vi "Main.vi"() -> ()   [LabVIEW 2023]
uses:
  Control/Time.ctl
panel:
  in  "stop":bool
  out "ms":dbl
  in  "碼表":bool
  in  "時鐘":bool
  in  "Tab Control":enum32{"Page 1", "Page 2"}(tab)
  out "Alarm Photo":picture
  out "Needle":cluster{dbl[], dbl[]}[](graph)
  out "clock":picture
  out "TIme":T1
  in  "Set Time":bool
  in  "Set second":i32(knob) scale=0.0..60.0
  in  "Set minute":i32(knob) scale=0.0..60.0
  in  "Set hour":i32(knob) scale=0.0..24.0
  in  "Set Alarm":bool
  in  "鬧鐘時間":timestamp format="%<%H:%M>T"
  in  "鬧鐘模式":u16(ring) items=["聲音模式", "畫面模式"]
  in  "Alarm Sound Path":path
  in  "Alarm Photo Path":path
  in  "開始/暫停碼表":bool
  in  "重置碼表":bool
  out "碼表時間":dbl
  out "碼表":i16(knob) scale=0.0..60.0
  out "smile":picture
  out "pi/180":dbl
  # "時"
  # "分"
  # "秒"
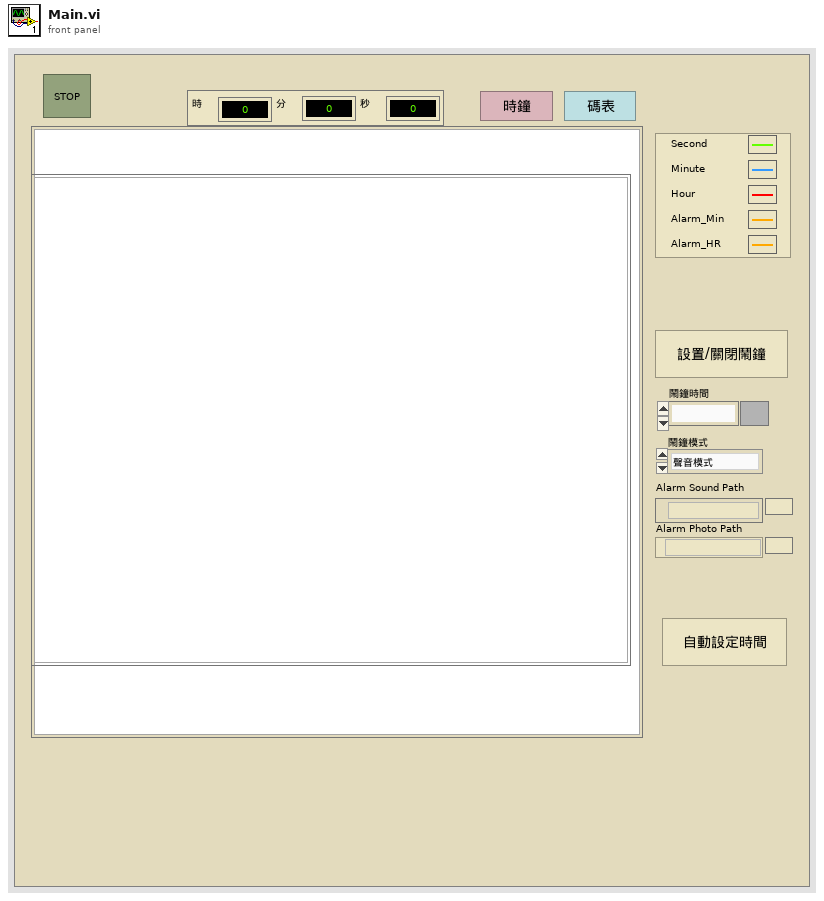
[diagram p1: front panel]
types:
  T1 = typedef "Time.ctl" = cluster{"hour":i32, "minute":i32, "second":i32}
  T2 = typedef "LVDateTimeRec.ctl" = cluster{"fractional second":dbl, "second":i32, "minute":i32, "hour":i32, "day of month":i32, "month":i32, "year":i32, "day of week":i32, "day of year":i32, "DST":i32}
  T3 = typedef "Sound Output Task ID.ctl" = u32
  T4 = typedef "imagedata.ctl" = cluster{"image type":i32, "image depth":i32, "image":u8[], "mask":u8[], "colors":u32[], "Rectangle":cluster{"left":i16, "top":i16, "right":i16, "bottom":i16}}
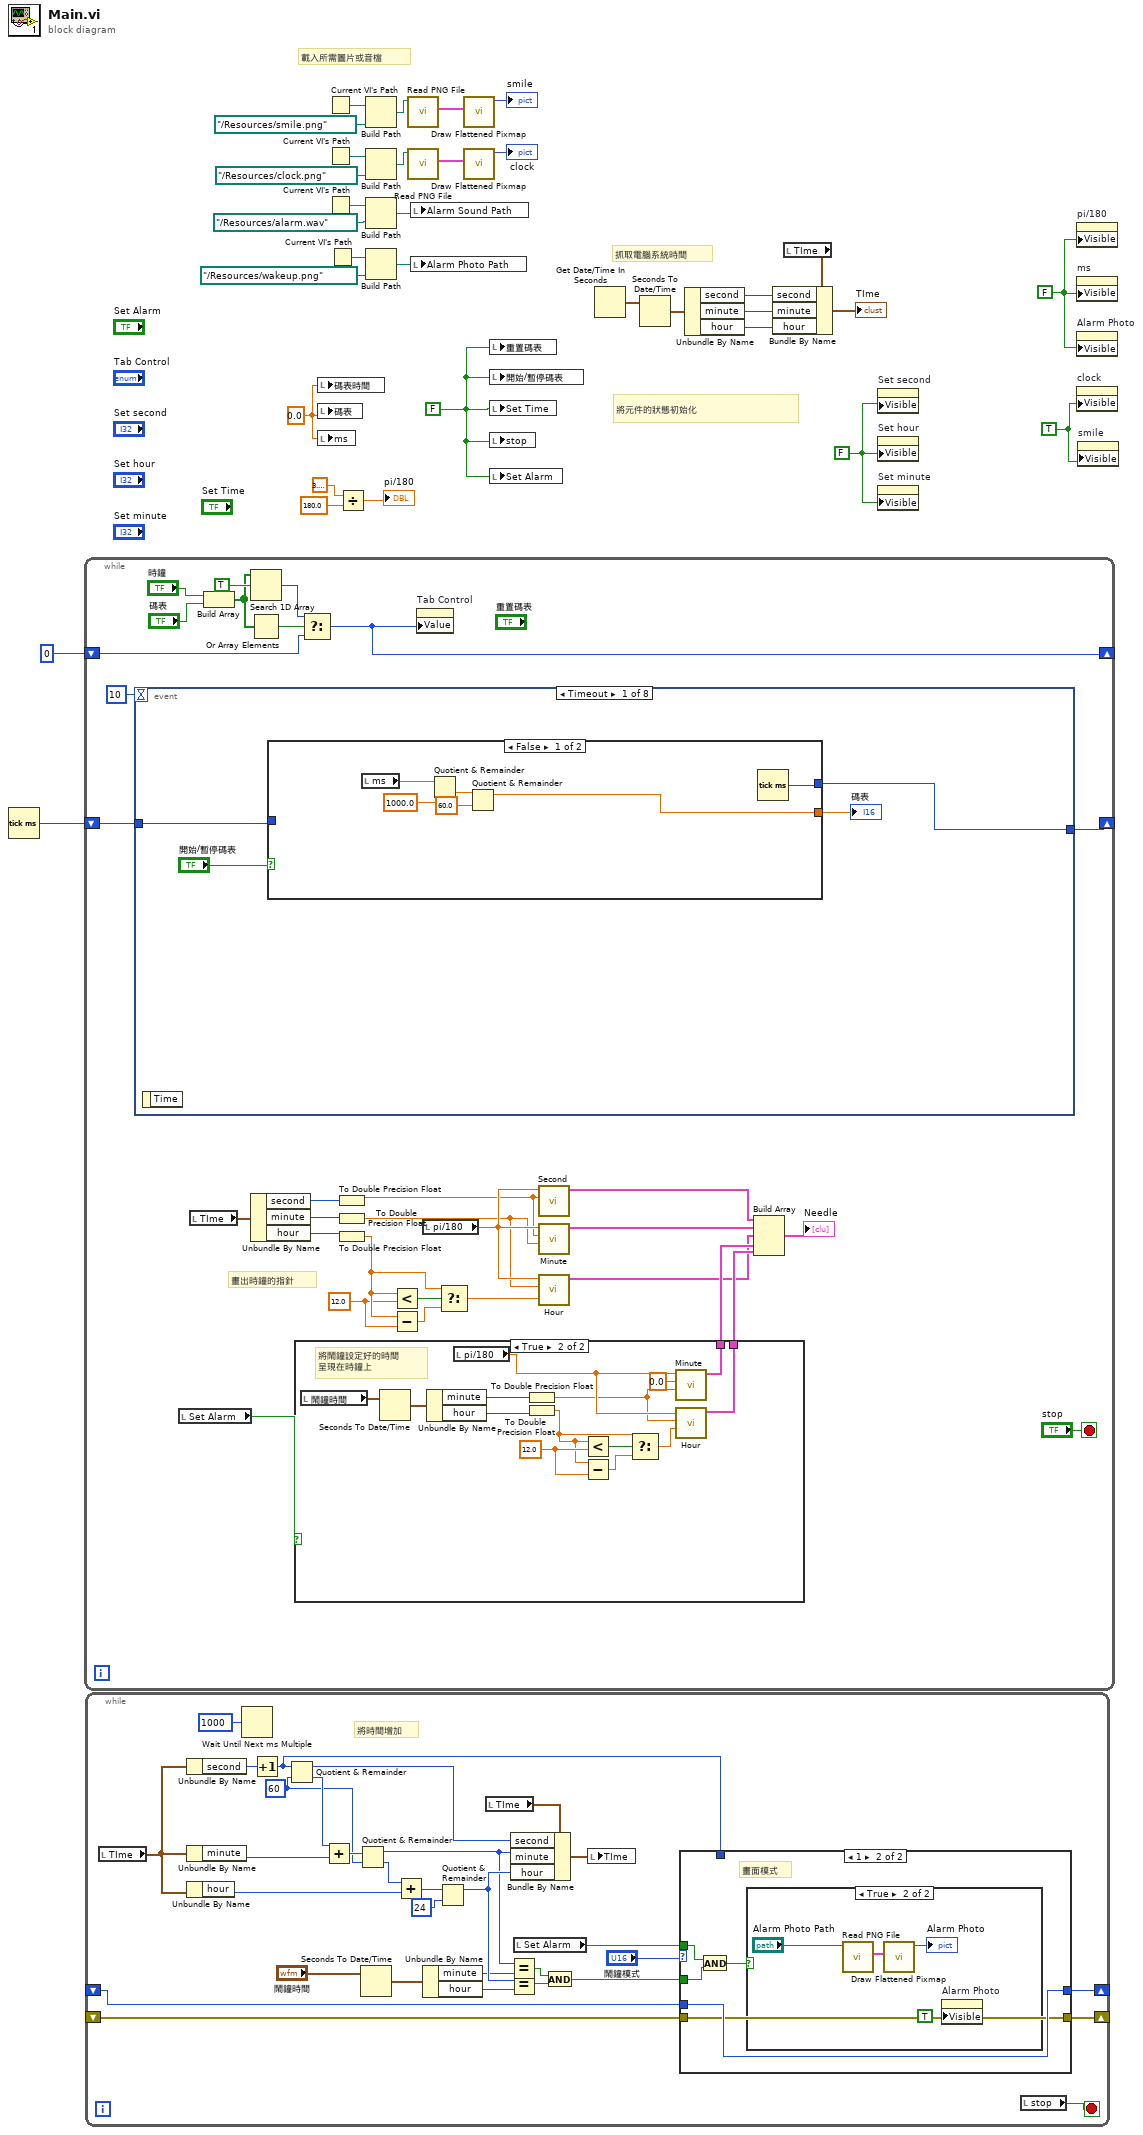
[diagram p0: block diagram]
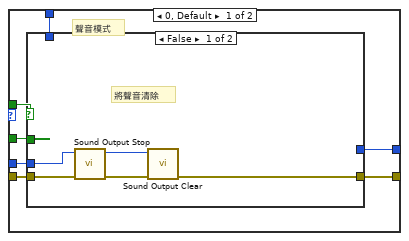
[diagram p2: hidden frame]
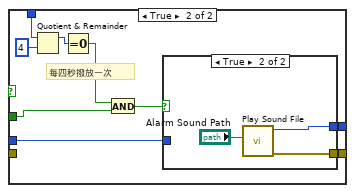
[diagram p3: hidden frame]
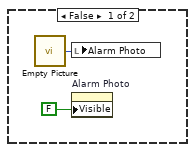
[diagram p5: hidden frame]
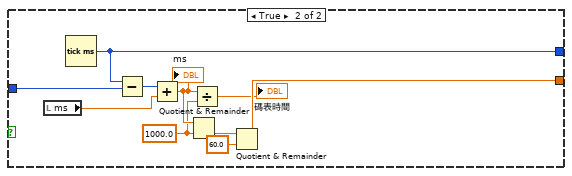
[diagram p7: hidden frame]
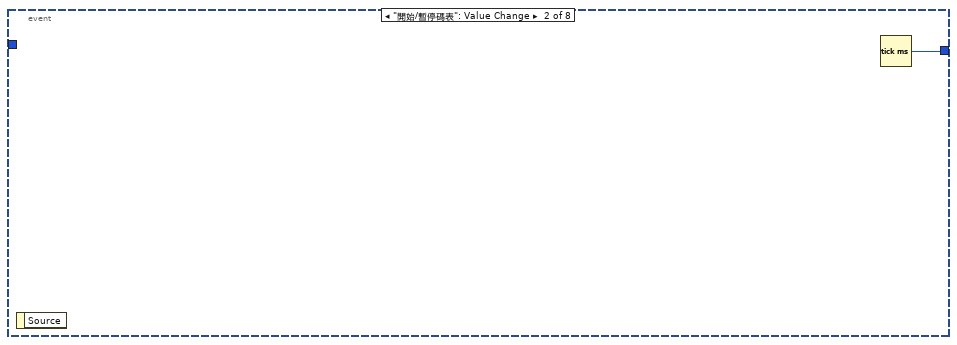
[diagram p8: hidden frame]
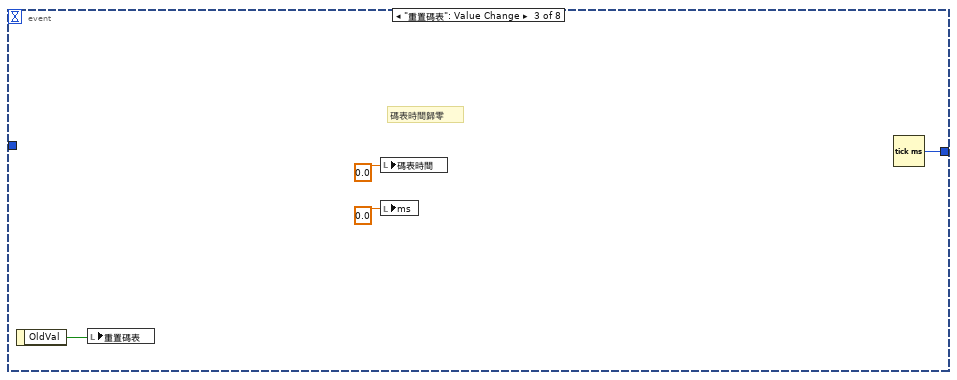
[diagram p9: hidden frame]
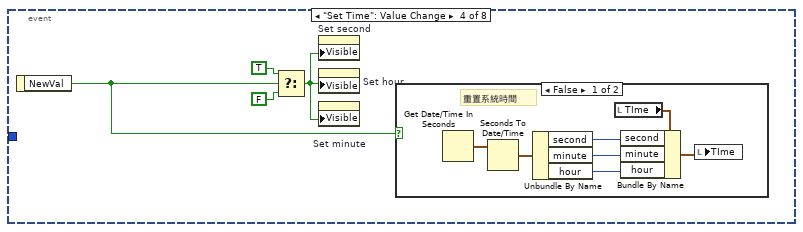
[diagram p10: hidden frame]
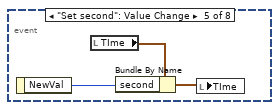
[diagram p12: hidden frame]
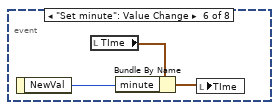
[diagram p13: hidden frame]
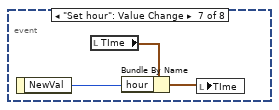
[diagram p14: hidden frame]
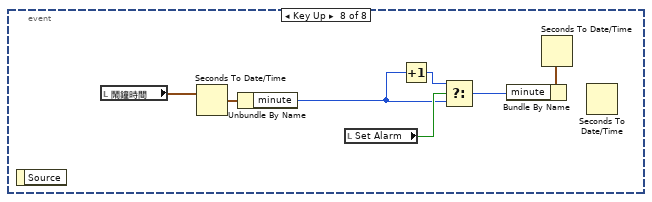
[diagram p15: hidden frame]
diagram:
  w1 = FALSE ("Visible")
  w2 = FALSE ("Visible")
  w10 = 0.0 ("碼表時間")
  w3 = TRUE
  w12 = FALSE ("Set time")
  # "將元件的狀態初始化"
  # "載入所需圖片或音檔"
  # "抓取電腦系統時間"
  n1 = Tick Count (ms)() -> (millisecond timer value=w11:u32)
  n2 = while {
    shift-right: [w55] -> _
    shift-left: 0 -> [w56]
    shift-right: [w53] -> _
    shift-left: w11 -> [w54]
    stop <- "stop" stop-if-true
    w34 = 12.0
    # "畫出時鐘的指針"
    n3 = event shown="[0] Timeout" {
      selector: _ -> [_ _ _ _ _ _ _ _]
      dyn-events: _ -> [_ _ _ _ _ _ _ _]
      timeout: 10 -> [_ _ _ _ _ _ _ _]
      tunnel: w54 -> [w81 _ _ _ _ _ _ _]
      tunnel: [w80 w99 w100 _ _ _ _ _] -> w53
      event Timeout {
        n4 = event-data() -> ()  [unwired: 1 in, 1 out]
        n5 = case shown="False" "開始/暫停碼表" {
          tunnel: [w85 w95] -> w79
          tunnel: w81 -> [_ w90]
          tunnel: [w83 w89] -> w80
          frame False {
            n6 = local read "ms"() -> (w84:dbl)
            n7 = Quotient & Remainder(x=w84, y=1000.0) -> (floor(x/y)=w88:dbl)  [unwired: 1 out]
            n8 = Quotient & Remainder(x=w88, y=60.0) -> (x-y*floor(x/y)=w85:dbl)  [unwired: 1 out]
            n9 = Tick Count (ms)() -> (millisecond timer value=w83:u32)
          }
          frame True {
            w93 = 1000.0 ("y")
            n10 = local read "ms"() -> (w91:dbl)
            n11 = Tick Count (ms)() -> (millisecond timer value=w89:u32)
            n12 = Subtract(x=w89, y=w90) -> (x-y=w97:u32)
            n13 = Add(x=w97, y=w91) -> (x+y=w94:dbl)
            "ms" <- w94
            n14 = Quotient & Remainder(x=w94, y=w93) -> (floor(x/y)=w98:dbl)  [unwired: 1 out]
            n15 = Divide(x=w94, y=w93) -> (x/y=→"碼表時間":dbl)
            n16 = Quotient & Remainder(x=w98, y=60.0) -> (x-y*floor(x/y)=w95:dbl)  [unwired: 1 out]
          }
        }
        "碼表" <- w79
      }
      event "開始/暫停碼表": Value Change {
        n17 = event-data() -> ()  [unwired: 1 in, 1 out]
        n18 = Tick Count (ms)() -> (millisecond timer value=w99:u32)
      }
      event "重置碼表": Value Change {
        # "碼表時間歸零"
        n19 = event-data() -> ("OldVal"=w103:bool)  [unwired: 1 in]
        n20 = local write "重置碼表"(w103) -> ()
        n21 = local write "碼表時間"(0.0 ("碼表時間")) -> ()
        n22 = local write "ms"(0.0 ("ms")) -> ()
        n23 = Tick Count (ms)() -> (millisecond timer value=w100:u32)
      }
      event "Set Time": Value Change {
        n24 = event-data() -> ("NewVal"=w107:bool)  [unwired: 1 in]
        n25 = Select(t=TRUE, s=w107, f=FALSE) -> (s? t:f=w104:bool)
        n26 = property on="Set second" class="Knob (strict)"("Visible"=w104) -> ()  [unwired: 2 in, 2 out]
        n27 = property on="Set hour" class="Knob (strict)"("Visible"=w104) -> ()  [unwired: 2 in, 2 out]
        n28 = property on="Set minute" class="Knob (strict)"("Visible"=w104) -> ()  [unwired: 2 in, 2 out]
        n29 = case shown="False" w107 {
          frame False {
            # "重置系統時間"
            n30 = Get Date/Time In Seconds() -> (seconds since 1Jan1904=w110:timestamp)
            n31 = Seconds To Date/Time(time stamp (now)=w110) -> (date time rec=w111:T2)  [unwired: 1 in]
            n32 = Unbundle By Name(w111) -> ("second"=w112:i32, "minute"=w113:i32, "hour"=w114:i32)
            n33 = local read "TIme"() -> (w109:T1)
            n34 = Bundle By Name(cluster=w109, "second"=w112, "minute"=w113, "hour"=w114) -> (w108:T1)
            n35 = local write "TIme"(w108) -> ()
          }
          frame True {
          }
        }
      }
      event "Set second": Value Change {
        n36 = event-data() -> ("NewVal"=w116:i32)  [unwired: 1 in]
        n37 = local read "TIme"() -> (w117:T1)
        n38 = Bundle By Name(cluster=w117, "second"=w116) -> (w115:T1)
        n39 = local write "TIme"(w115) -> ()
      }
      event "Set minute": Value Change {
        n40 = event-data() -> ("NewVal"=w119:i32)  [unwired: 1 in]
        n41 = local read "TIme"() -> (w120:T1)
        n42 = Bundle By Name(cluster=w120, "minute"=w119) -> (w118:T1)
        n43 = local write "TIme"(w118) -> ()
      }
      event "Set hour": Value Change {
        n44 = event-data() -> ("NewVal"=w122:i32)  [unwired: 1 in]
        n45 = local read "TIme"() -> (w123:T1)
        n46 = Bundle By Name(cluster=w123, "hour"=w122) -> (w121:T1)
        n47 = local write "TIme"(w121) -> ()
      }
      event Key Up {
        n48 = event-data() -> ()  [unwired: 1 in, 1 out]
        n49 = local read "鬧鐘時間"() -> (w128:timestamp)
        n50 = Seconds To Date/Time(time stamp (now)=w128) -> (date time rec=w127:T2)  [unwired: 1 in]
        n51 = Unbundle By Name(w127) -> ("minute"=w126:i32)
        n52 = local read "Set Alarm"() -> (w129:bool)
        n53 = Increment(x=w126) -> (x+1=w130:i32)
        n54 = Select(t=w130, s=w129, f=w126) -> (s? t:f=w124:i32)
        n55 = Seconds To Date/Time() -> (date time rec=w125:T2)  [unwired: 2 in]
        n56 = Bundle By Name(cluster=w125, "minute"=w124) -> ()  [unwired: 1 out]
        n57 = Seconds To Date/Time() -> ()  [unwired: 2 in, 1 out]
      }
    }
    n58 = local read "Set Alarm"() -> (w48:bool)
    n59 = local read "TIme"() -> (w46:T1)
    n60 = Build Array("時鐘", "碼表") -> (w59:bool[])
    n61 = Search 1D Array(1D array=w59, element=TRUE) -> (index of element=w57:i32)  [unwired: 1 in]
    n62 = Or Array Elements(Boolean array=w59) -> (logical OR=w58:bool)
    n63 = Unbundle By Name(w46) -> ("second"=w47:i32, "minute"=w49:i32, "hour"=w50:i32)
    n64 = case shown="True" w48 {
      tunnel: [_ w69] -> w51
      tunnel: [_ w68] -> w52
      frame False {
        # "沒有設定鬧鐘的話就傳空的"
      }
      frame True {
        w75 = 12.0
        # "將鬧鐘設定好的時間\n呈現在時鐘上"
        n65 = local read "鬧鐘時間"() -> (w77:timestamp)
        n66 = Seconds To Date/Time(time stamp (now)=w77) -> (date time rec=w78:T2)  [unwired: 1 in]
        n67 = Unbundle By Name(w78) -> ("minute"=w66:i32, "hour"=w65:i32)
        n68 = local read "pi/180"() -> (w76:dbl)
        n69 = To Double Precision Float(number=w66) -> (double precision float=w71:dbl)
        n70 = To Double Precision Float(number=w65) -> (double precision float=w67:dbl)
        n71 = Less?(x=w67, y=w75) -> (x < y?=w74:bool)
        n72 = Subtract(x=w67, y=w75) -> (x-y=w73:dbl)
        n73 = Select(t=w67, s=w74, f=w73) -> (s? t:f=w72:dbl)
        n74 = call "Minute.vi"("Minute"=w71, "Second"=0.0, "pi/180"=w76) -> ("Cluster"=w69:cluster{dbl[], dbl[]})  [unwired: 8 in]
        n75 = call "Hour.vi"("Hour"=w72, "Minute"=w71, "pi/180"=w76) -> ("Cluster"=w68:cluster{dbl[], dbl[]})  [unwired: 8 in]
      }
    }
    n76 = Select(t=w57, s=w58, f=w56) -> (s? t:f=w55:i32)
    n77 = To Double Precision Float(number=w47) -> (double precision float=w40:dbl)
    n78 = To Double Precision Float(number=w49) -> (double precision float=w39:dbl)
    n79 = To Double Precision Float(number=w50) -> (double precision float=w37:dbl)
    n80 = Less?(x=w37, y=w34) -> (x < y?=w35:bool)
    n81 = Subtract(x=w37, y=w34) -> (x-y=w36:dbl)
    n82 = property on="Tab Control" class="TabCtl (strict)"("Value"=w55) -> ()  [unwired: 2 in, 2 out]
    n83 = local read "pi/180"() -> (w45:dbl)
    n84 = Select(t=w37, s=w35, f=w36) -> (s? t:f=w38:dbl)
    n85 = call "Second.vi"("Numeric"=w40, "pi/180"=w45) -> ("Cluster"=w41:cluster{dbl[], dbl[]})  [unwired: 9 in]
    n86 = call "Minute.vi"("Minute"=w39, "Second"=w40, "pi/180"=w45) -> ("Cluster"=w42:cluster{dbl[], dbl[]})  [unwired: 8 in]
    n87 = call "Hour.vi"("Hour"=w38, "Minute"=w39, "pi/180"=w45) -> ("Cluster"=w43:cluster{dbl[], dbl[]})  [unwired: 8 in]
    n88 = Build Array(w41, w42, w43, w51, w52) -> (→"Needle":cluster{dbl[], dbl[]}[])
  }
  n89 = while {
    shift-right: [w144] -> _
    shift-left: _ -> [w142]
    shift-right: [w145] -> _
    shift-left: _ -> [w143]
    stop <- w148 stop-if-true
    w151 = 60 ("y")
    # "將時間增加"
    n90 = local read "TIme"() -> (w161:T1)
    n91 = Unbundle By Name(w161) -> ("second"=w160:i32)
    n92 = Unbundle By Name(w161) -> ("minute"=w159:i32)
    n93 = Unbundle By Name(w161) -> ("hour"=w156:i32)
    n94 = Wait Until Next ms Multiple(millisecond multiple=u32 1000) -> ()  [unwired: 1 out]
    n95 = Increment(x=w160) -> (x+1=w132:i32)
    n96 = Quotient & Remainder(x=w132, y=w151) -> (x-y*floor(x/y)=w134:i32, floor(x/y)=w158:i32)
    n97 = Add(x=w158, y=w159) -> (x+y=w157:i32)
    n98 = Quotient & Remainder(x=w157, y=w151) -> (x-y*floor(x/y)=w139:i32, floor(x/y)=w155:i32)
    n99 = Seconds To Date/Time(time stamp (now)="鬧鐘時間") -> (date time rec=w146:T2)  [unwired: 1 in]
    n100 = Add(x=w155, y=w156) -> (x+y=w154:i32)
    n101 = Unbundle By Name(w146) -> ("minute"=w135:i32, "hour"=w136:i32)
    n102 = Quotient & Remainder(x=w154, y=24) -> (x-y*floor(x/y)=w140:i32)  [unwired: 1 out]
    n103 = local read "TIme"() -> (w150:T1)
    n104 = Equal?(x=w139, y=w135) -> (x = y?=w138:bool)
    n105 = Equal?(x=w140, y=w136) -> (x = y?=w137:bool)
    n106 = Bundle By Name(cluster=w150, "second"=w134, "minute"=w139, "hour"=w140) -> (w149:T1)
    n107 = local read "Set Alarm"() -> (w141:bool)
    n108 = And(x=w138, y=w137) -> (x .and. y?=w133:bool)
    n109 = local write "TIme"(w149) -> ()
    n110 = case shown="1" "鬧鐘模式" {
      tunnel: [w168 w191] -> w145
      tunnel: [w167 w190] -> w144
      tunnel: w143 -> [w166 w191]
      tunnel: w142 -> [w165 w190]
      tunnel: w141 -> [w164 w188]
      tunnel: w133 -> [w163 w187]
      tunnel: w132 -> [w162 _]
      frame 0, Default {
        # "聲音模式"
        n111 = case shown="False" w164 {
          tunnel: [_ w182] -> w168
          tunnel: [w169 w181] -> w167
          tunnel: w166 -> [w173 w180]
          tunnel: w165 -> [w171 _]
          tunnel: w163 -> [_ w176]
          tunnel: w162 -> [_ w175]
          frame False {
            # "將聲音清除"
            n112 = call <vilib>:"Sound Output Stop.vi"("error in (no error)"=w171, "task ID"=w173) -> ("error out"=w170:errorcluster, "task ID out"=w172:T3)  [unwired: 8 in]
            n113 = call <vilib>:"Sound Output Clear.vi"("error in (no error)"=w170, "task ID"=w172) -> ("error out"=w169:errorcluster)  [unwired: 9 in]
          }
          frame True {
            # "每四秒撥放一次"
            n114 = Quotient & Remainder(x=w175, y=4) -> (x-y*floor(x/y)=w174:i32)  [unwired: 1 out]
            n115 = Equal To 0?(x=w174) -> (x = 0?=w177:bool)
            n116 = And(x=w177, y=w176) -> (x .and. y?=w178:bool)
            n117 = case shown="True" w178 {
              tunnel: [w183 w185] -> w182
              tunnel: [_ w184] -> w181
              tunnel: w180 -> [w183 _]
              frame False {
              }
              frame True {
                n118 = call <vilib>:"Play Sound File.vi"("path"="Alarm Sound Path") -> ("error out"=w184:errorcluster, "task ID"=w185:T3)  [unwired: 9 in]
              }
            }
          }
        }
      }
      frame 1 {
        # "畫面模式"
        n119 = And(x=w188, y=w187) -> (x .and. y?=w189:bool)
        n120 = case shown="True" w189 {
          frame False {
            n121 = call "Empty Picture"() -> ("empty picture"=w193:picture)
            n122 = local write "Alarm Photo"(w193) -> ()
            n123 = property on="Alarm Photo" class="Pict"("Visible"=FALSE) -> ()  [unwired: 2 in, 2 out]
          }
          frame True {
            n124 = call <vilib>:"Read PNG File.vi"("path to PNG file"="Alarm Photo Path") -> ("image data"=w196:T4)  [unwired: 8 in, 2 out]
            n125 = call <vilib>:"Draw Flattened Pixmap.vi"("image data"=w196) -> ("new picture"=→"Alarm Photo":picture)  [unwired: 8 in]
            n126 = property on="Alarm Photo" class="Pict"("Visible"=TRUE) -> ()  [unwired: 2 in, 2 out]
          }
        }
      }
    }
    n127 = local read "stop"() -> (w148:bool)
  }
  n128 = local write "碼表時間"(w10) -> ()
  n129 = local write "碼表"(w10) -> ()
  n130 = local write "ms"(w10) -> ()
  n131 = Current VI's Path() -> (path=w8:path)
  n132 = Current VI's Path() -> (path=w33:path)
  n133 = Current VI's Path() -> (path=w14:path)
  n134 = Current VI's Path() -> (path=w18:path)
  n135 = Divide(x=3.141592653589793, y=180.0) -> (x/y=→"pi/180":dbl)
  n136 = Build Path(base path=w8, name or relative path=path "../Resources/smile.png") -> (appended path=w6:path)
  n137 = Build Path(base path=w33, name or relative path=path "../Resources/clock.png") -> (appended path=w9:path)
  n138 = Build Path(base path=w14, name or relative path=path "../Resources/alarm.wav") -> (appended path=w19:path)
  n139 = Build Path(base path=w18, name or relative path=path "../Resources/wakeup.png") -> (appended path=w16:path)
  n140 = call <vilib>:"Read PNG File.vi"("path to PNG file"=w6) -> ("image data"=w5:T4)  [unwired: 8 in, 2 out]
  n141 = call <vilib>:"Read PNG File.vi"("path to PNG file"=w9) -> ("image data"=w31:T4)  [unwired: 8 in, 2 out]
  n142 = local write "Alarm Sound Path"(w19) -> ()
  n143 = local write "Alarm Photo Path"(w16) -> ()
  n144 = call <vilib>:"Draw Flattened Pixmap.vi"("image data"=w5) -> ("new picture"=→"smile":picture)  [unwired: 8 in]
  n145 = call <vilib>:"Draw Flattened Pixmap.vi"("image data"=w31) -> ("new picture"=→"clock":picture)  [unwired: 8 in]
  n146 = local write "重置碼表"(w12) -> ()
  n147 = local write "開始/暫停碼表"(w12) -> ()
  n148 = local write "Set Time"(w12) -> ()
  n149 = local write "stop"(w12) -> ()
  n150 = local write "Set Alarm"(w12) -> ()
  n151 = Get Date/Time In Seconds() -> (seconds since 1Jan1904=w26:timestamp)
  n152 = Seconds To Date/Time(time stamp (now)=w26) -> (date time rec=w25:T2)  [unwired: 1 in]
  n153 = Unbundle By Name(w25) -> ("second"=w24:i32, "minute"=w23:i32, "hour"=w22:i32)
  n154 = local read "TIme"() -> (w20:T1)
  n155 = Bundle By Name(cluster=w20, "second"=w24, "minute"=w23, "hour"=w22) -> (→"TIme":T1)
  n156 = property on="Set second" class="Knob (strict)"("Visible"=w1) -> ()  [unwired: 2 in, 2 out]
  n157 = property on="Set hour" class="Knob (strict)"("Visible"=w1) -> ()  [unwired: 2 in, 2 out]
  n158 = property on="Set minute" class="Knob (strict)"("Visible"=w1) -> ()  [unwired: 2 in, 2 out]
  n159 = property on="pi/180" class="DigNum (strict)"("Visible"=w2) -> ()  [unwired: 2 in, 2 out]
  n160 = property on="ms" class="DigNum (strict)"("Visible"=w2) -> ()  [unwired: 2 in, 2 out]
  n161 = property on="Alarm Photo" class="Pict"("Visible"=w2) -> ()  [unwired: 2 in, 2 out]
  n162 = property on="clock" class="Pict"("Visible"=w3) -> ()  [unwired: 2 in, 2 out]
  n163 = property on="smile" class="Pict"("Visible"=w3) -> ()  [unwired: 2 in, 2 out]
